vi "Calculate UV In Pixels.vi"(7 "Texture Dimensions":T2, 11 "UV":T3 {"v" min=0 max=1 step=0.1; "u" min=0 max=1 step=0.1}) -> (3 "Pixels":T1)   [LabVIEW 2022 SP3, in "Raster.lvlib"]
uses:
  Raster.lvlib
  UV.ctl
  Rectangle Dimensions.ctl
  Point 2D.ctl
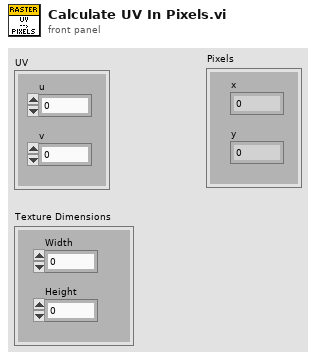
[diagram p1: front panel]
types:
  T1 = typedef "Raster.lvlib/Point 2D.ctl" = cluster{"x":i32, "y":i32}
  T2 = typedef "Raster.lvlib/Rectangle Dimensions.ctl" = cluster{"Width":u32, "Height":u32}
  T3 = typedef "Raster.lvlib/UV.ctl" = cluster{"u":sgl, "v":sgl}
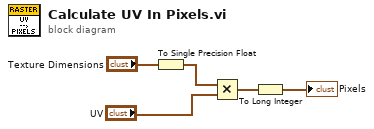
[diagram p0: block diagram]
diagram:
  n1 = To Single Precision Float(number="Texture Dimensions") -> (single precision float=w4:cluster{"Width":sgl, "Height":sgl})
  n2 = Multiply(x=w4, y="UV") -> (x*y=w2:T3)
  n3 = To Long Integer(number=w2) -> (32bit integer=→"Pixels":cluster{"u":i32, "v":i32})
